vi "Autonomous Independent.vi"   [LabVIEW 2017]
doc: "This VI is called when autonomous begins, and will automatically be terminated when autonomous ends. You can carry out timed or sensor driven robot movement independently without needing to return to the caller."
uses:
  <vilib>/Rock Robotics/WPI/Utilities/WPI_GetSetVariantRefNum.vi
  <vilib>/Rock Robotics/Network Tables/NT Read String.vi
  <vilib>/Rock Robotics/WPI/RobotDrive/WPI_RobotDriveMecanumDrive_Cartesian.vi
  <vilib>/Rock Robotics/Network Tables/NT Write Numeric Array.vi
panel:
  # "Be sure to right-click and choose Data Operations>>Make Current Value default if you want to save the array values with the VI"
types:
  T1 = typedef "WPI_JoystickDevRef.ctl" = cluster{"Device":T2}
  T2 = typedef "WPI_JoystickDeviceEnum.ctl" = enum16{"USB 0", "USB 1", "USB 2", "USB 3", "USB 4", "USB 5"}
  T3 = typedef "WPI_RobotDriveDevRef.ctl" = cluster{"DevStatus":errorcluster, "Motors[]":T4[], "Square Inputs":bool, "Max Output":dbl}
  T4 = typedef "WPI_MotorControlDeviceRef.ctl" = cluster{"DeviceStatus":errorcluster, "Type":T5, "PWM":cluster{"PWM Channel":T6, "DeadBand":T7}, "CAN":cluster{"Device Number":u8, "SetOutput VI Ref":variant, "GetOutput VI Ref":variant, "Enable VI Ref":variant, "Disable VI Ref":variant, "Data":variant}, "Invert":bool, "DIO PWM":cluster{"PWM \"Enable\" Channel":T6, "DIOChannel":T8, "PWM Rate":dbl}}
  T5 = typedef "WPI_MotorControlType.ctl" = enum16{"PWM", "CAN", "DIO PWM"}
  T6 = typedef "FPGA_DIOPWMChannel.ctl" = enum8{"PWM 0", "PWM 1", "PWM 2", "PWM 3", "PWM 4", "PWM 5", "PWM 6", "PWM 7", "PWM 8", "PWM 9", "PWM MXP 0", "PWM MXP 1", "PWM MXP 2", "PWM MXP 3", "PWM MXP 4", "PWM MXP 5", "PWM MXP 6", "PWM MXP 7", "PWM MXP 8", "PWM MXP 9", "Invalid"}
  T7 = typedef "WPI_PWMDeadband.ctl" = cluster{"Name":string, "maxPositivePwm":i32, "minPositivePwm":i32, "centerPwm":i32, "maxNegativePwm":i32, "minNegativePwm":i32, "angularRange":u16}
  T8 = typedef "FPGA_DIOChannel.ctl" = enum8{"DIO 0", "DIO 1", "DIO 2", "DIO 3", "DIO 4", "DIO 5", "DIO 6", "DIO 7", "DIO 8", "DIO 9", "DIO MXP 0", "DIO MXP 1", "DIO MXP 2", "DIO MXP 3", "DIO MXP 4", "DIO MXP 5", "DIO MXP 6", "DIO MXP 7", "DIO MXP 8", "DIO MXP 9", "DIO MXP 10", "DIO MXP 11", "DIO MXP 12", "DIO MXP 13", "DIO MXP 14", "DIO MXP 15", "SPI Port CS1", "SPI Port CS2", "SPI Port CS3", "SPI Port MISO", "SPI Port MOSI", "Invalid"}
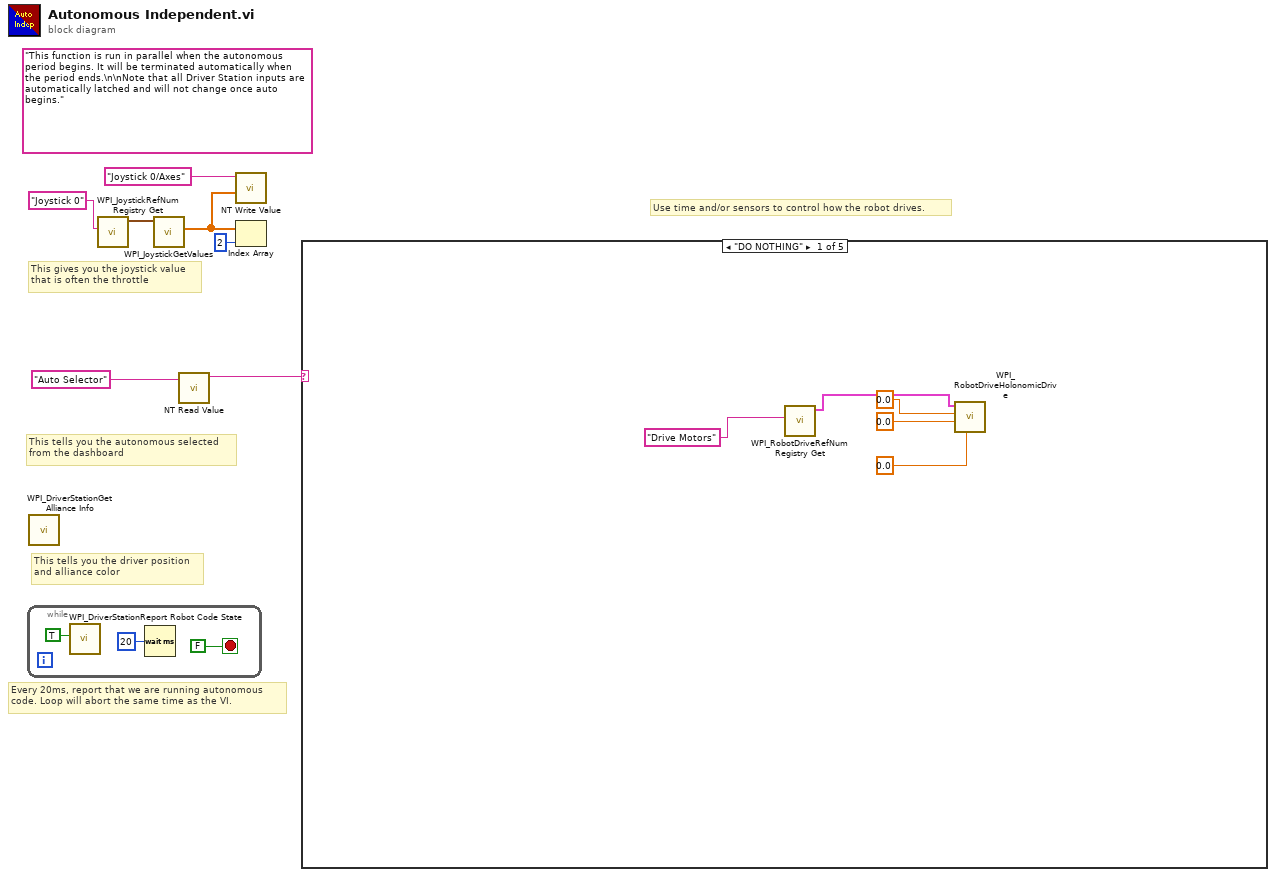
[diagram p0: block diagram]
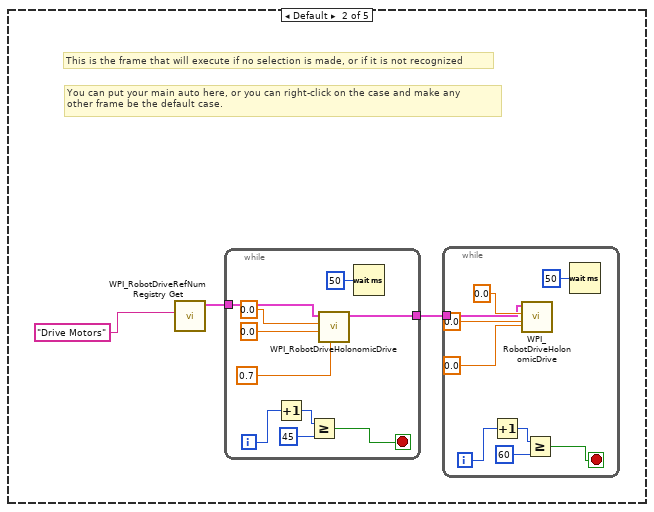
[diagram p2: hidden frame]
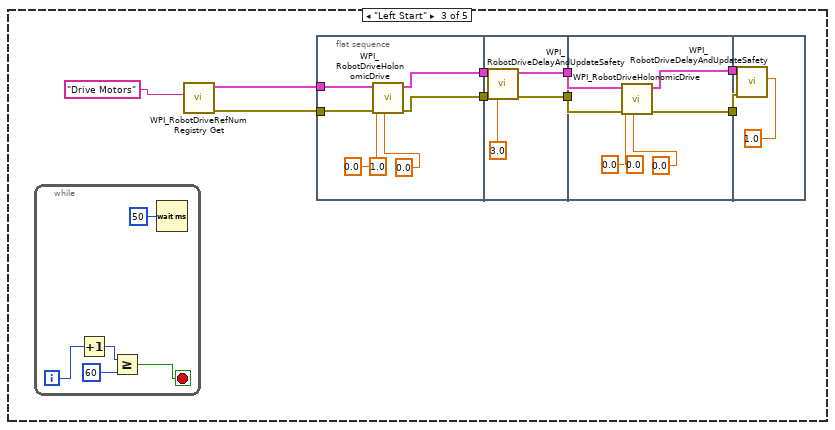
[diagram p3: hidden frame]
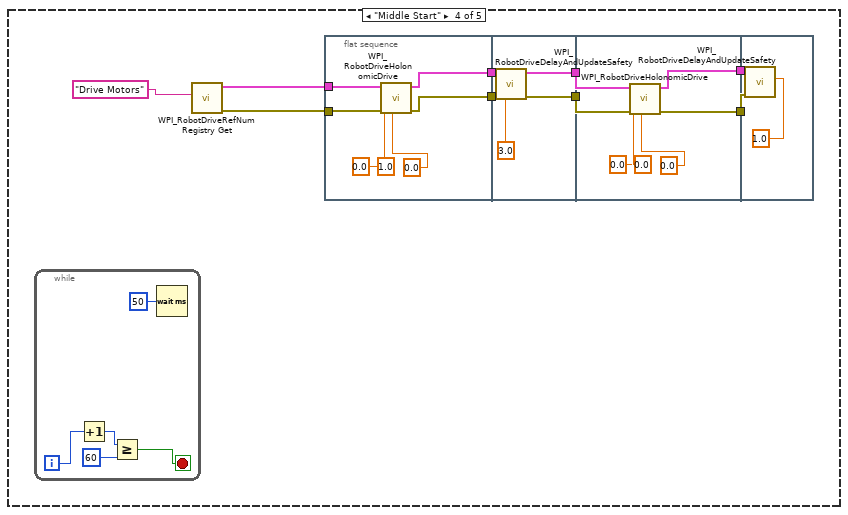
[diagram p4: hidden frame]
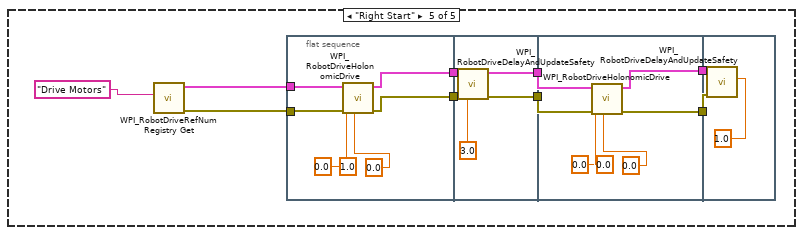
[diagram p5: hidden frame]
diagram:
  (unwired) "This function is run in parallel when the autonomous period begins. It will be terminated automatically when the period ends.\n\nNote that all Driver Station inputs are automatically latched and will not change once auto begins."
  # "This tells you the autonomous selected\nfrom the dashboard"
  # "Every 20ms, report that we are running autonomous\ncode. Loop will abort the same time as the VI."
  # "This gives you the joystick value\nthat is often the throttle"
  # "Use time and/or sensors to control how the robot drives."
  # "This tells you the driver position\nand alliance color"
  n1 = while {
    stop <- FALSE stop-if-true
    n2 = call <vilib>:"WPI_DriverStationReport Robot Code State.vi"("Autonomous"=TRUE) -> ()  [unwired: 10 in, 1 out]
    n3 = Wait (ms)(milliseconds to wait=u32 20) -> ()  [unwired: 1 out]
  }
  n4 = call <vilib>:"WPI_DriverStationGet Alliance Info.vi"() -> ()  [unwired: 12 out]
  n5 = call <vilib>:"WPI_JoystickRefNum Registry Get.vi"("refnum name"="Joystick 0") -> ("JoystickDevRef"=w6:T1)  [unwired: 1 in, 9 out]
  n6 = call <vilib>:"WPI_JoystickGetValues.vi"("JoystickDevRef"=w6) -> ("Axes"=w2:dbl[])  [unwired: 6 in, 4 out]
  n7 = call-poly <vilib>:"NT Read Value.vi"("Name"="Auto Selector") -> ("String"=w3:string)  [unwired: 9 in, 1 out]
  n8 = call-poly <vilib>:"NT Write Value.vi"("Numeric Array"=w2, "Name"="Joystick 0/Axes") -> ()  [unwired: 9 in, 1 out]
  n9 = Index Array(array=w2, index=2) -> ()  [unwired: 1 out]
  n10 = case shown="\"DO NOTHING\"" w3 {
    frame "DO NOTHING" {
      n11 = call <vilib>:"WPI_RobotDriveRefNum Registry Get.vi"("refnum name"="Drive Motors") -> ("RobotDriveDevRef"=w11:T3)  [unwired: 9 in, 1 out]
      n12 = call-poly <vilib>:"WPI_RobotDriveHolonomicDrive.vi"("Rotation"=0.0, "Y"=0.0, "X"=0.0, "RobotDriveDevRef"=w11) -> ()  [unwired: 5 in, 3 out]
    }
    frame Default {
      # "You can put your main auto here, or you can right-click on the case and make any\nother frame be the default case."
      # "This is the frame that will execute if no selection is made, or if it is not recognized"
      n13 = call <vilib>:"WPI_RobotDriveRefNum Registry Get.vi"("refnum name"="Drive Motors") -> ("RobotDriveDevRef"=w17:T3)  [unwired: 9 in, 1 out]
      n14 = while {
        tunnel: w17 -> [w29]
        tunnel: [w28] -> w16
        i -> [w35]
        stop <- w36 stop-if-true
        n15 = Increment(x=w35) -> (x+1=w34:i32)
        n16 = Greater Or Equal?(x=w34, y=45) -> (x >= y?=w36:bool)
        n17 = call-poly <vilib>:"WPI_RobotDriveHolonomicDrive.vi"("Rotation"=0.7, "Y"=0.0, "X"=0.0, "RobotDriveDevRef"=w29) -> ("RobotDriveDevRef"=w28:T3)  [unwired: 5 in, 2 out]
        n18 = Wait (ms)(milliseconds to wait=u32 50) -> ()  [unwired: 1 out]
      }
      n19 = while {
        tunnel: w16 -> [w19]
        i -> [w25]
        stop <- w26 stop-if-true
        n20 = Increment(x=w25) -> (x+1=w24:i32)
        n21 = call-poly <vilib>:"WPI_RobotDriveHolonomicDrive.vi"("Rotation"=0.0, "Y"=0.0, "X"=0.0, "RobotDriveDevRef"=w19) -> ()  [unwired: 5 in, 3 out]
        n22 = Greater Or Equal?(x=w24, y=60) -> (x >= y?=w26:bool)
        n23 = Wait (ms)(milliseconds to wait=u32 50) -> ()  [unwired: 1 out]
      }
    }
    frame "Left Start" {
      n24 = while {
        i -> [w49]
        stop <- w50 stop-if-true
        n25 = Increment(x=w49) -> (x+1=w48:i32)
        n26 = Greater Or Equal?(x=w48, y=60) -> (x >= y?=w50:bool)
        n27 = Wait (ms)(milliseconds to wait=u32 50) -> ()  [unwired: 1 out]
      }
      n28 = call <vilib>:"WPI_RobotDriveRefNum Registry Get.vi"("refnum name"="Drive Motors") -> ("error out"=w39:errorcluster, "RobotDriveDevRef"=w40:T3)  [unwired: 9 in]
      n29 = flat-sequence {
        tunnel: [w55] -> w46
        tunnel: [w54] -> w45
        tunnel: w39 -> [w53]
        tunnel: w40 -> [w52]
        tunnel: w46 -> [w63]
        tunnel: w45 -> [w62]
        tunnel: [w61] -> w44
        tunnel: [w60] -> w43
        tunnel: w44 -> [w69]
        tunnel: w43 -> [w66]
        tunnel: [w65] -> w42
        tunnel: [w64] -> w41
        tunnel: w42 -> [w73]
        tunnel: w41 -> [w71]
        frame #0 {
          n30 = call-poly <vilib>:"WPI_RobotDriveHolonomicDrive.vi"("Rotation"=0.0, "error in (no error)"=w53, "Y"=1.0, "X"=0.0, "RobotDriveDevRef"=w52) -> ("error out"=w55:errorcluster, "RobotDriveDevRef"=w54:T3)  [unwired: 4 in, 1 out]
        }
        frame #1 {
          n31 = call <vilib>:"WPI_RobotDriveDelayAndUpdateSafety.vi"("error in (no error)"=w63, "Delay (s)"=3.0, "RobotDriveDevRef"=w62) -> ("error out"=w61:errorcluster, "RobotDriveDevRef 2"=w60:T3)  [unwired: 7 in]
        }
        frame #2 {
          n32 = call-poly <vilib>:"WPI_RobotDriveHolonomicDrive.vi"("Rotation"=0.0, "error in (no error)"=w69, "Y"=0.0, "X"=0.0, "RobotDriveDevRef"=w66) -> ("error out"=w65:errorcluster, "RobotDriveDevRef"=w64:T3)  [unwired: 4 in, 1 out]
        }
        frame #3 {
          n33 = call <vilib>:"WPI_RobotDriveDelayAndUpdateSafety.vi"("error in (no error)"=w73, "Delay (s)"=1.0, "RobotDriveDevRef"=w71) -> ()  [unwired: 7 in, 2 out]
        }
      }
    }
    frame "Middle Start" {
      n34 = while {
        i -> [w85]
        stop <- w86 stop-if-true
        n35 = Increment(x=w85) -> (x+1=w84:i32)
        n36 = Greater Or Equal?(x=w84, y=60) -> (x >= y?=w86:bool)
        n37 = Wait (ms)(milliseconds to wait=u32 50) -> ()  [unwired: 1 out]
      }
      n38 = call <vilib>:"WPI_RobotDriveRefNum Registry Get.vi"("refnum name"="Drive Motors") -> ("error out"=w75:errorcluster, "RobotDriveDevRef"=w74:T3)  [unwired: 9 in]
      n39 = flat-sequence {
        tunnel: [w91] -> w82
        tunnel: [w90] -> w81
        tunnel: w75 -> [w89]
        tunnel: w74 -> [w88]
        tunnel: w82 -> [w99]
        tunnel: w81 -> [w98]
        tunnel: [w97] -> w80
        tunnel: [w96] -> w79
        tunnel: w80 -> [w105]
        tunnel: w79 -> [w102]
        tunnel: [w101] -> w78
        tunnel: [w100] -> w77
        tunnel: w78 -> [w109]
        tunnel: w77 -> [w107]
        frame #0 {
          n40 = call-poly <vilib>:"WPI_RobotDriveHolonomicDrive.vi"("Rotation"=0.0, "error in (no error)"=w89, "Y"=1.0, "X"=0.0, "RobotDriveDevRef"=w88) -> ("error out"=w91:errorcluster, "RobotDriveDevRef"=w90:T3)  [unwired: 4 in, 1 out]
        }
        frame #1 {
          n41 = call <vilib>:"WPI_RobotDriveDelayAndUpdateSafety.vi"("error in (no error)"=w99, "Delay (s)"=3.0, "RobotDriveDevRef"=w98) -> ("error out"=w97:errorcluster, "RobotDriveDevRef 2"=w96:T3)  [unwired: 7 in]
        }
        frame #2 {
          n42 = call-poly <vilib>:"WPI_RobotDriveHolonomicDrive.vi"("Rotation"=0.0, "error in (no error)"=w105, "Y"=0.0, "X"=0.0, "RobotDriveDevRef"=w102) -> ("error out"=w101:errorcluster, "RobotDriveDevRef"=w100:T3)  [unwired: 4 in, 1 out]
        }
        frame #3 {
          n43 = call <vilib>:"WPI_RobotDriveDelayAndUpdateSafety.vi"("error in (no error)"=w109, "Delay (s)"=1.0, "RobotDriveDevRef"=w107) -> ()  [unwired: 7 in, 2 out]
        }
      }
    }
    frame "Right Start" {
      n44 = call <vilib>:"WPI_RobotDriveRefNum Registry Get.vi"("refnum name"="Drive Motors") -> ("error out"=w111:errorcluster, "RobotDriveDevRef"=w110:T3)  [unwired: 9 in]
      n45 = flat-sequence {
        tunnel: [w122] -> w118
        tunnel: [w121] -> w117
        tunnel: w111 -> [w120]
        tunnel: w110 -> [w119]
        tunnel: w118 -> [w130]
        tunnel: w117 -> [w129]
        tunnel: [w128] -> w116
        tunnel: [w127] -> w115
        tunnel: w116 -> [w136]
        tunnel: w115 -> [w133]
        tunnel: [w132] -> w114
        tunnel: [w131] -> w113
        tunnel: w114 -> [w140]
        tunnel: w113 -> [w138]
        frame #0 {
          n46 = call-poly <vilib>:"WPI_RobotDriveHolonomicDrive.vi"("Rotation"=0.0, "error in (no error)"=w120, "Y"=1.0, "X"=0.0, "RobotDriveDevRef"=w119) -> ("error out"=w122:errorcluster, "RobotDriveDevRef"=w121:T3)  [unwired: 4 in, 1 out]
        }
        frame #1 {
          n47 = call <vilib>:"WPI_RobotDriveDelayAndUpdateSafety.vi"("error in (no error)"=w130, "Delay (s)"=3.0, "RobotDriveDevRef"=w129) -> ("error out"=w128:errorcluster, "RobotDriveDevRef 2"=w127:T3)  [unwired: 7 in]
        }
        frame #2 {
          n48 = call-poly <vilib>:"WPI_RobotDriveHolonomicDrive.vi"("Rotation"=0.0, "error in (no error)"=w136, "Y"=0.0, "X"=0.0, "RobotDriveDevRef"=w133) -> ("error out"=w132:errorcluster, "RobotDriveDevRef"=w131:T3)  [unwired: 4 in, 1 out]
        }
        frame #3 {
          n49 = call <vilib>:"WPI_RobotDriveDelayAndUpdateSafety.vi"("error in (no error)"=w140, "Delay (s)"=1.0, "RobotDriveDevRef"=w138) -> ()  [unwired: 7 in, 2 out]
        }
      }
    }
  }
